vi "Get Random Eat Sound.vi"(8 "error in (no error)":errorcluster, 11 "Application in":refnum<class "Application.lvclass">) -> (0 "error out":errorcluster, 3 "Random Eat Sound":path)   [LabVIEW 2021, in "Application.lvclass"]
uses:
  Application.lvclass
  Application.lvclass/Application.ctl
  <vilib>/numeric/Random Number (Range) U64.vi
  <vilib>/numeric/sub_Random U32.vi
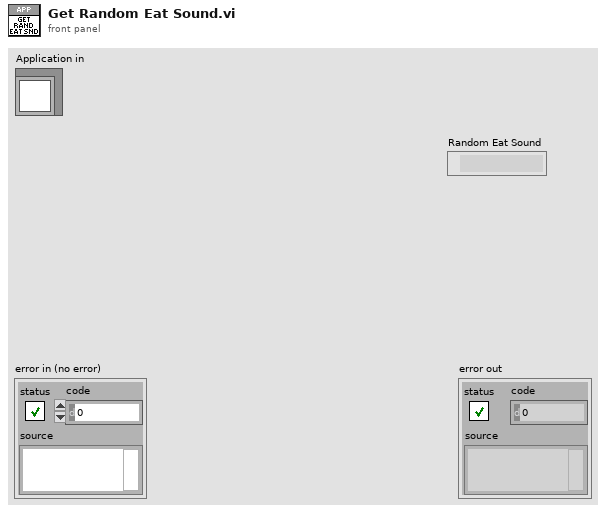
[diagram p1: front panel]
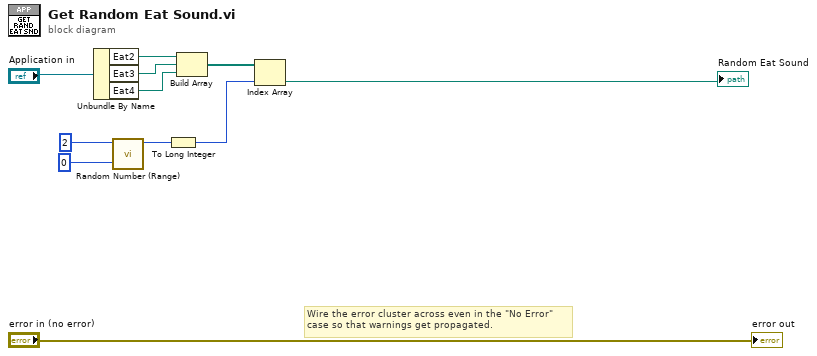
[diagram p0: block diagram]
diagram:
  # "Wire the error cluster across even in the \"No Error\"\ncase so that warnings get propagated."
  n1 = Unbundle By Name("Application in") -> ("Eat2"=w7:path, "Eat3"=w6:path, "Eat4"=w5:path)
  n2 = call-poly <vilib>:"Random Number (Range).vi"("lower bound (0)"=u64 0, "upper bound (100)"=u64 2) -> ("number"=w3:u64)  [unwired: 9 in]
  n3 = To Long Integer(number=w3) -> (32bit integer=w2:i32)
  n4 = Build Array(w7, w6, w5) -> (w4:path[])
  n5 = Index Array(array=w4, index=w2) -> (element=→"Random Eat Sound":path)
  "error out" <- "error in (no error)"
